vi "TCP Write (Asynchronous) - Byte Array.vi"(8 "error in":errorcluster, 9 "Timeout ms (default 50ms)":i32=50, 10 "Unsigned Byte Array":u8[](array[numeric]), 11 "TCP Network Connection in":refnum<k5>) -> (0 "error out":errorcluster, 3 "TCP Network Connection out":refnum<k5>)   [LabVIEW 2017, in "Communications Library.lvlib"]
doc: "Writes a byte array to a TCP port."
uses:
  Communications Library.lvlib
  Error 5102 - DTACQ unit replied with an error--const.vi
  <vilib>/Utility/error.llb/Error Cluster From Error Code.vi
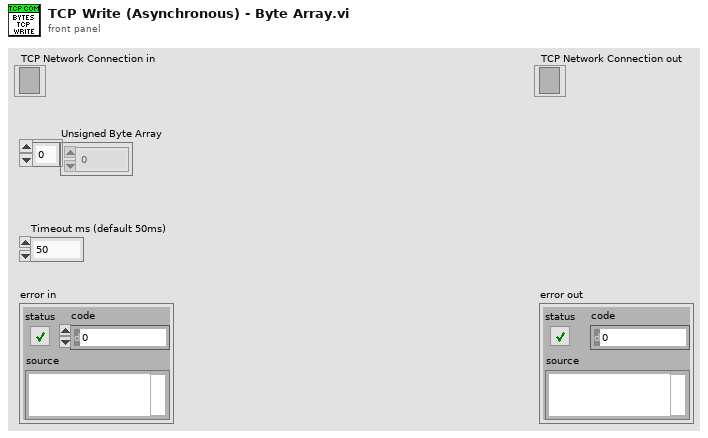
[diagram p1: front panel]
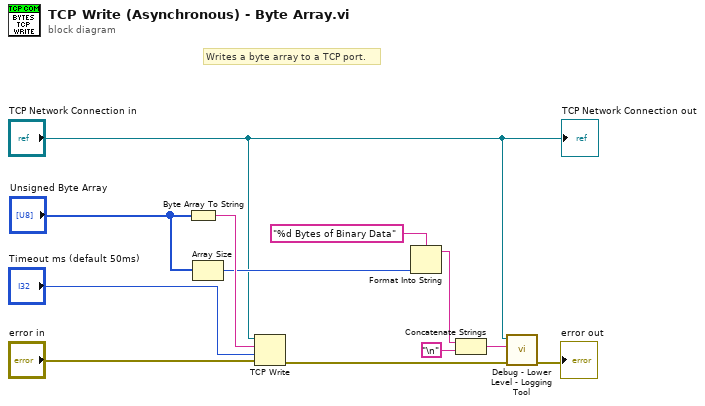
[diagram p0: block diagram]
diagram:
  # "Writes a byte array to a TCP port."
  n1 = Byte Array To String(unsigned byte array="Unsigned Byte Array") -> (string=w11:string)
  n2 = Array Size(array="Unsigned Byte Array") -> (size(s)=w9:i32)
  n3 = TCP Write(connection ID="TCP Network Connection in", data in=w11, error in (no error)="error in", 9:"Timeout ms (default 50ms)") -> (error out=w7:errorcluster)  [unwired: 2 out]
  n4 = Format Into String(format string="%d Bytes of Binary Data", w9) -> (resulting string=w1:string)  [unwired: 2 in, 1 out]
  n5 = Concatenate Strings(w1, "\n") -> (w2:string)
  n6 = call "Debug - Lower Level - Logging Tool.vi"("Error In"=w7, "Data Sent"=w2, "TCP Network Connecion In"="TCP Network Connection in") -> ("Error Out"=→"error out":errorcluster)  [unwired: 7 in, 1 out]
  "TCP Network Connection out" <- "TCP Network Connection in"
